vi "Get Node Children.vi"(10 "Type Definitions":refnum<vi>, 11 "Node Name":string) -> (3 "Children":string[](array[string]))   [LabVIEW 2025]
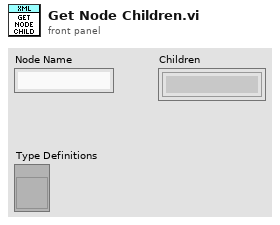
[diagram p1: front panel]
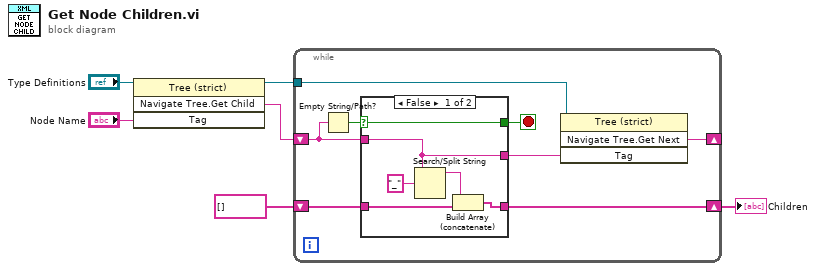
[diagram p0: block diagram]
diagram:
  n1 = invoke on="Invoke Node" class="Tree (strict)" method="Navigate Tree.Get Child"(reference="Type Definitions", "Tag"="Node Name") -> (reference out=w2:refnum<vi>, "Navigate Tree:Get Child"=w4:string)  [unwired: 2 in, 2 out]
  n2 = while {
    shift-right: [w12] -> w3
    shift-left: string[] [] -> [w13]
    shift-right: [w10] -> _
    shift-left: w4 -> [w8]
    tunnel: w2 -> [w9]
    stop <- w14 stop-if-true
    n3 = Empty String/Path?(string/path=w8) -> (empty?=w7:bool)
    n4 = case shown="False" w7 {
      selector: w7 -> [w15 w22]
      tunnel: [w15 w22] -> w14
      tunnel: w13 -> [w19 w21]
      tunnel: [w20 w21] -> w12
      tunnel: w8 -> [w17 _]
      tunnel: [w17 _] -> w11
      frame False {
        n5 = Search/Split String(string=w17, search string/char (-)="_") -> (substring before match=w18:string)  [unwired: 1 in, 2 out]
        n6 = Build Array (concatenate)(w18, w19) -> (w20:string[])
      }
      frame True {
      }
    }
    n7 = invoke on="Invoke Node" class="Tree (strict)" method="Navigate Tree.Get Next"(reference=w9, "Tag"=w11) -> ("Navigate Tree:Get Next Item"=w10:string)  [unwired: 2 in, 3 out]
  }
  "Children" <- w3
